vi "sub_sample_without_replacement.vi"(8 "error in (no error)":errorcluster, 9 "number of unique samples":i32, 10 "probability":dbl[](array[numeric]), 11 "List":i32[](array[numeric])=[0, 0, 0, 0, 0, 0, 0, 0, 0, 0]) -> (0 "error out":errorcluster, 2 "probability not equal to 1":bool, 3 "unique samples":i32[](array[numeric]))   [LabVIEW 2021]
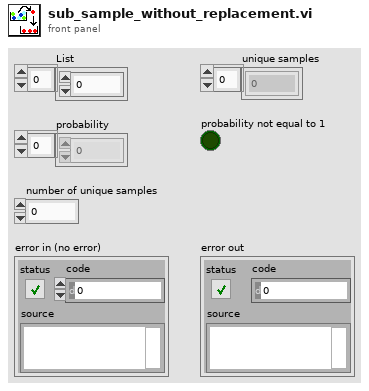
[diagram p1: front panel]
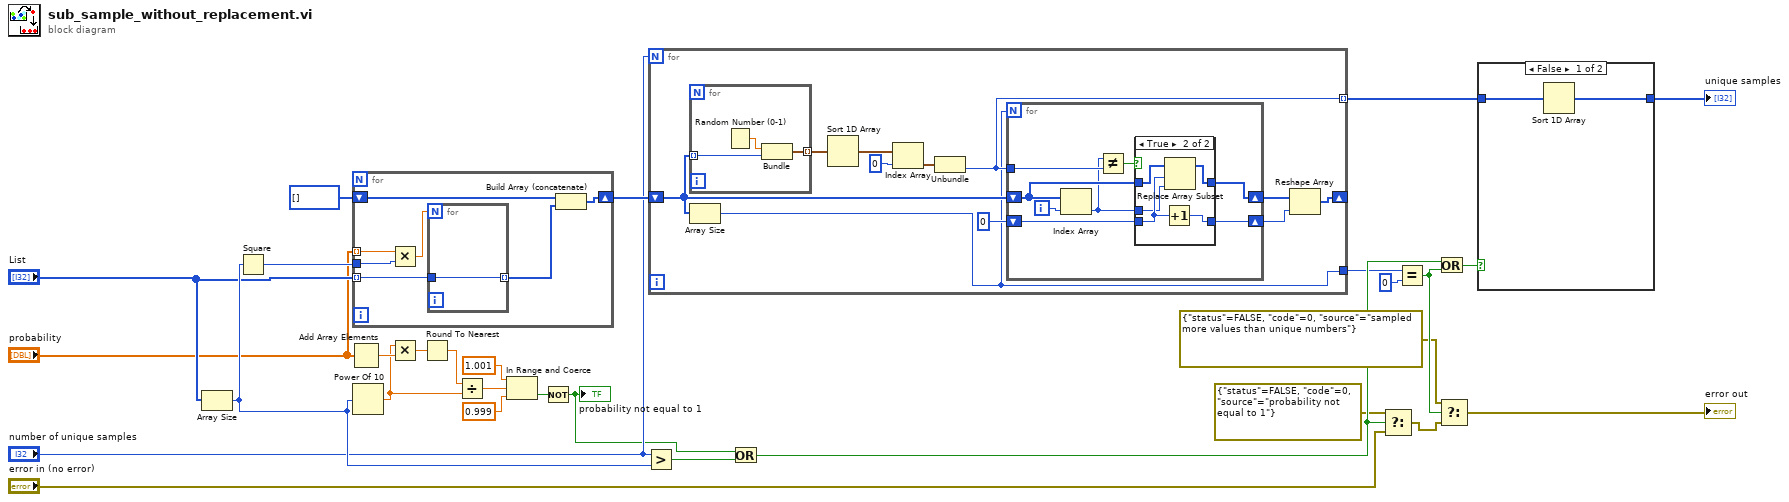
[diagram p0: block diagram]
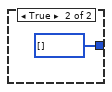
[diagram p2: hidden frame]
diagram:
  n1 = Array Size(array="List") -> (size(s)=w16:i32)
  n2 = Square(x=w16) -> (x^2=w12:i32)
  n3 = Add Array Elements(numeric array="probability") -> (sum=w11:dbl)
  n4 = for {
    tunnel: "probability" -> [w36] mode=indexing
    tunnel: "List" -> [w34] mode=indexing
    shift-right: [w32] -> w19
    shift-left: i32[] [] -> [w31]
    tunnel: w12 -> [w30]
    n5 = Multiply(x=w36, y=w30) -> (x*y=w35:dbl)
    n6 = for {
      N: w35 -> [_]
      tunnel: w34 -> [w37]
      tunnel: [w37] -> w33 mode=indexing
    }
    n7 = Build Array (concatenate)(w31, w33) -> (w32:i32[])
  }
  n8 = Power Of 10(x=w16) -> (10^x=w10:dbl)
  n9 = Multiply(x=w10, y=w11) -> (x*y=w8:dbl)
  n10 = Round To Nearest(number=w8) -> (nearest integer value=w9:dbl)
  n11 = Divide(x=w9, y=w10) -> (x/y=w5:dbl)
  n12 = In Range and Coerce(upper limit=1.001, x=w5, lower limit=0.999) -> (In Range?=w2:bool)  [unwired: 1 out]
  n13 = Not(x=w2) -> (.not. x?=w1:bool)
  "probability not equal to 1" <- w1
  n14 = Greater?(x="number of unique samples", y=w16) -> (0:w17:bool)
  n15 = for {
    N: "number of unique samples" -> [_]
    tunnel: [w41] -> w26 mode=indexing
    shift-right: [w40] -> _
    shift-left: w19 -> [w39]
    tunnel: [w38] -> w22
    n16 = for {
      tunnel: [w66] -> w48 mode=indexing
      tunnel: w39 -> [w64] mode=indexing
      n17 = Random Number (0-1)() -> (number: 0 to 1=w65:dbl)
      n18 = Bundle("number: 0 to 1"=w65, w64) -> (w66:cluster{"number: 0 to 1":dbl, i32})  [unwired: 1 out]
    }
    n19 = Array Size(array=w39) -> (size(s)=w38:i32)
    n20 = Sort 1D Array(array=w48) -> (sorted array=w47:cluster{"number: 0 to 1":dbl, i32}[])
    n21 = Index Array(array=w47, index=0) -> (element=w46:cluster{"number: 0 to 1":dbl, i32})
    n22 = Unbundle(w46) -> (w41:i32)  [unwired: 1 out]
    n23 = for {
      N: w38 -> [_]
      shift-right: [w56] -> w43
      shift-left: w39 -> [w54]
      shift-right: [w52] -> w42
      shift-left: 0 -> [w53]
      tunnel: w41 -> [w51]
      i -> [w55]
      n24 = Index Array(array=w54, index=w55) -> (element=w49:i32)
      n25 = Not Equal?(x=w49, y=w51) -> (x != y?=w50:bool)
      n26 = case shown="True" w50 {
        tunnel: w54 -> [w58 w63]
        tunnel: [w58 w62] -> w56
        tunnel: w53 -> [w57 w61]
        tunnel: [w57 w60] -> w52
        tunnel: w49 -> [_ w59]
        frame False {
        }
        frame True {
          n27 = Increment(x=w61) -> (x+1=w60:i32)
          n28 = Replace Array Subset(array=w63, new element=w59, index=w61) -> (w62:i32[])
        }
      }
    }
    n29 = Reshape Array(w43, w42) -> (w40:i32[])
  }
  n30 = Or(x=w1, y=w17) -> (x .or. y?=w27:bool)
  n31 = Select(t=errorcluster {"status"=FALSE, "code"=0, "source"="probability not equal to 1"} ("error constant"), s=w27, f="error in (no error)") -> (s? t:f=w24:errorcluster)
  n32 = Equal?(x=w22, y=0) -> (x = y?=w28:bool)
  n33 = Or(x=w27, y=w28) -> (x .or. y?=w29:bool)
  n34 = Select(t=errorcluster {"status"=FALSE, "code"=0, "source"="sampled more values than unique numbers"} ("error constant"), s=w28, f=w24) -> (s? t:f=→"error out":errorcluster)
  n35 = case shown="False" w29 {
    tunnel: [w67 i32[] []] -> w25
    tunnel: w26 -> [w68 _]
    frame False {
      n36 = Sort 1D Array(array=w68) -> (sorted array=w67:i32[])
    }
    frame True {
    }
  }
  "unique samples" <- w25
